vi "CCM-Save Table.vi"(0 "configuration file path":path=path "C:/PXI Connections.txt", 2 "IO Type":T2, 5 "Table":T1[](array[typedef]), 9 "Endpoints":cluster{"Items":string[]}, 11 "error in (no error)":errorcluster) -> (4 "file path":path, 15 "error out":errorcluster)   [LabVIEW 2020]
uses:
  Type Defs/CM-IO Type.ctl
  Type Defs/CM-Connection.ctl
  <vilib>/Utility/config.llb/Write Key (String).vi
  <vilib>/Utility/config.llb/NI_LVConfig.lvlib
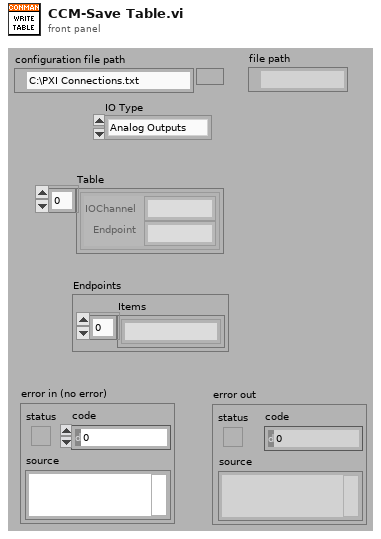
[diagram p1: front panel]
types:
  T1 = typedef "CM-Connection.ctl" = cluster{"IOChannel":string, "Endpoint":string}
  T2 = typedef "CM-IO Type.ctl" = enum16{"Analog Outputs", "Analog Inputs", "Digital Outputs", "Digital Inputs"}
  T3 = typedef "NI_LVConfig.lvlib/Config Data RefNum.ctl" = refnum<k1>
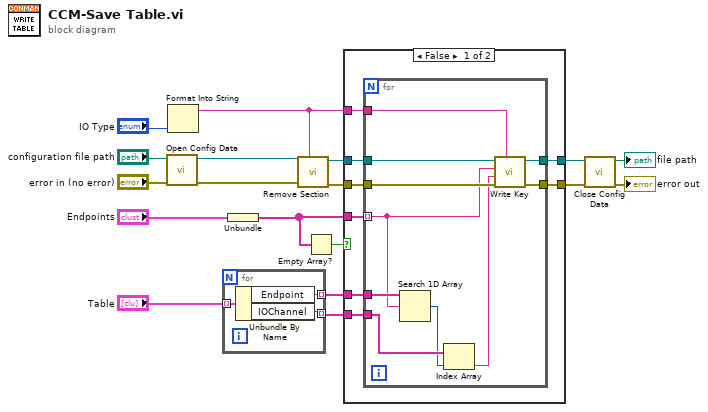
[diagram p0: block diagram]
diagram:
  n1 = call <vilib>:"Open Config Data.vi"("error in (no error)"="error in (no error)", "configuration file path"="configuration file path") -> ("error out"=w14:errorcluster, "refnum"=w15:T3)  [unwired: 7 in, 1 out]
  n2 = Format Into String("IO Type") -> (resulting string=w3:string)  [unwired: 3 in, 1 out]
  n3 = for {
    tunnel: "Table" -> [w21] mode=indexing
    tunnel: [w20] -> w7 mode=indexing
    tunnel: [w19] -> w6 mode=indexing
    n4 = Unbundle By Name(w21) -> ("Endpoint"=w20:string, "IOChannel"=w19:string)
  }
  n5 = Unbundle("Endpoints") -> ("Items"=w5:string[])
  n6 = call <vilib>:"Remove Section.vi"("section"=w3, "error in (no error)"=w14, "refnum"=w15) -> ("error out"=w8:errorcluster, "refnum out"=w9:T3)  [unwired: 6 in, 1 out]
  n7 = Empty Array?(array=w5) -> (empty?=w10:bool)
  n8 = case shown="False" w10 {
    tunnel: w7 -> [w29 _]
    tunnel: w9 -> [w28 w41]
    tunnel: w8 -> [w27 w40]
    tunnel: w5 -> [w26 _]
    tunnel: [w25 w41] -> w13
    tunnel: [w24 w40] -> w12
    tunnel: w3 -> [w23 _]
    tunnel: w6 -> [w22 _]
    frame False {
      n9 = for {
        tunnel: w26 -> [w34] mode=indexing
        tunnel: w29 -> [w39]
        tunnel: w28 -> [w38]
        tunnel: [w36] -> w25
        tunnel: w27 -> [w37]
        tunnel: [w35] -> w24
        tunnel: w23 -> [w33]
        tunnel: w22 -> [w32]
        n10 = Search 1D Array(1D array=w39, element=w34) -> (index of element=w31:i32)  [unwired: 1 in]
        n11 = Index Array(array=w32, index=w31) -> (element=w30:string)
        n12 = call-poly <vilib>:"Write Key.vi"("section"=w33, "error in (no error)"=w37, "value"=w30, "key"=w34, "refnum"=w38) -> ("error out"=w35:errorcluster, "refnum out"=w36:T3)  [unwired: 4 in, 1 out]
      }
    }
    frame True {
    }
  }
  n13 = call <vilib>:"Close Config Data.vi"("error in (no error)"=w12, "refnum"=w13) -> ("error out"=→"error out":errorcluster, "file path"=→"file path":path)  [unwired: 8 in]
